vi "Command Response.vi"(8 "error in (no error)":errorcluster, 10 "Message":refnum<class "Message Interface.lvclass">, 11 "Controller in":refnum<class "Controller.lvclass">) -> (0 "error out":errorcluster, 3 "Controller out":refnum<class "Controller.lvclass">)   [LabVIEW 2016, in "Controller Actor.lvlib" / "Controller.lvclass"]
uses:
  <userlib>/Common Components/Controller/Controller.lvclass
  <userlib>/Composed Systems/Stream/Mediator/Classes/Message Interface/Message Interface.lvclass
  <userlib>/Composed Systems/Stream/Mediator/Classes/Websocket Message Broker Interface Ref/Websocket Message Broker Interface Ref.lvclass/Websocket Message Broker Interface Ref.ctl
  <userlib>/Common Components/WebSocket Networking/WS Message Broker Interface Ref/WS Message Broker Interface Ref.lvclass
  C:/Program Files (x86)/National Instruments/LabVIEW 2016/user.lib/Composed Systems/Stream/Mediator/Classes/Websocket Message Broker Interface Ref/Websocket Message Broker Interface Ref.lvclass
  <userlib>/Composed Systems/Stream/Mediator/Classes/Message Transport Queue/Message Transport Queue.lvclass
  <userlib>/Common Components/WebSocket Networking/WS Server Msgs/WSserver Command Response Msg/WSserver Command Response Msg.lvclass
  <userlib>/Composed Systems/Stream/Mediator/Classes/Websocket Message Broker Interface Ref/Websocket Message Broker Interface Ref.lvclass
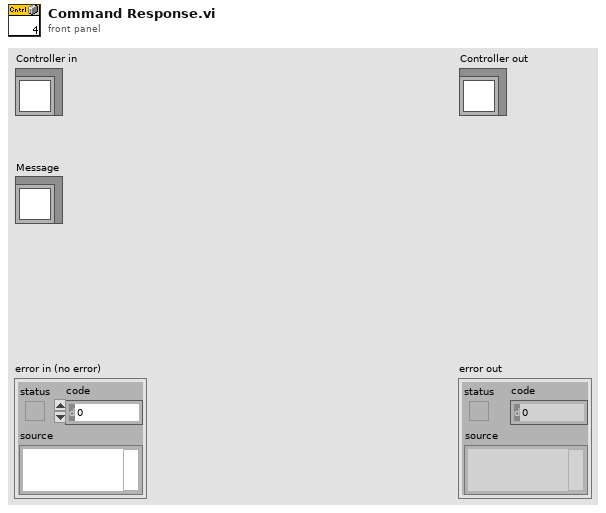
[diagram p1: front panel]
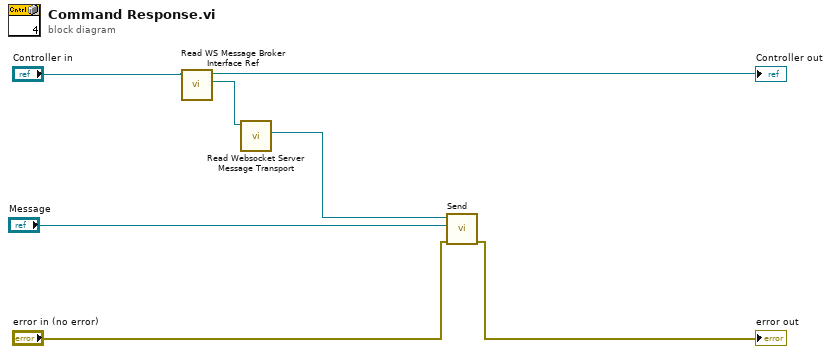
[diagram p0: block diagram]
diagram:
  n1 = call-dynamic "Read WS Message Broker Interface Ref.vi"("Controller in"="Controller in") -> ("WS Message Broker Interface Ref.lvclass"=w4:refnum<class "WS Message Broker Interface Ref.lvclass">, "Controller out"=→"Controller out":refnum<class "Controller.lvclass">)  [unwired: 9 in]
  n2 = call <userlib>:"Read Websocket Server Message Transport.vi"("Websocket Message Broker Interface Ref in"=w4) -> ("Stream Mediator.lvlib:Message Transport Queue.lvclass"=w3:refnum<class "Message Transport Queue.lvclass">)  [unwired: 9 in, 1 out]
  n3 = call <userlib>:"Send.vi"("error in (no error)"="error in (no error)", "Message"="Message", "Message Transport Queue"=w3) -> ("error out"=→"error out":errorcluster)  [unwired: 8 in]
